vi "CommandLine.vi"() -> ()   [LabVIEW 2009]
doc: "This example shows how to use Command Line Arguments property node to launch a LabVIEW VI and pass user-defined arguments.\n\nUse the following syntax in the Command Line to launch this VI:\n\n\"<full path to LabVIEW directory>\\labview.exe\" \"<full path to LabVIEW directory>\\examples\\viserver\\cmdline.llb\\CommandLine.vi\"\n\nThis will launch CommandLine.vi\n\nThis VI is set to run when opened.\n\nAfter the VI name, enter two hyphens (--) surrounded by spaces before the user-defined arguments. \n\nThe arguments will be displayed in the front panel indicators.\n\nThe correct syntax for arguments that can be passed is\n/number:\n/boolean:\n/string:\nAfter (:) enter the appropriate value; a number, 0 or 1 boolean, a string.\n\nIf you enter more than one argument, they need to be separated with a space."
uses:
  <vilib>/Utility/miscctls.llb/LVRectTypeDef.ctl
panel:
  out "Command Line Arguments":string[](array[string])
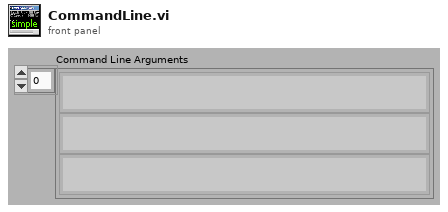
[diagram p1: front panel]
types:
  T1 = typedef "LVRectTypeDef.ctl" = cluster{"Left":i16, "Top":i16, "Right":i16, "Bottom":i16}
  T2 = enum16{"big-endian, network order", "native, host order", "little-endian"}
  T3 = enum16{"open", "replace", "create", "open or create", "replace or create", "replace or create with confirmation"}
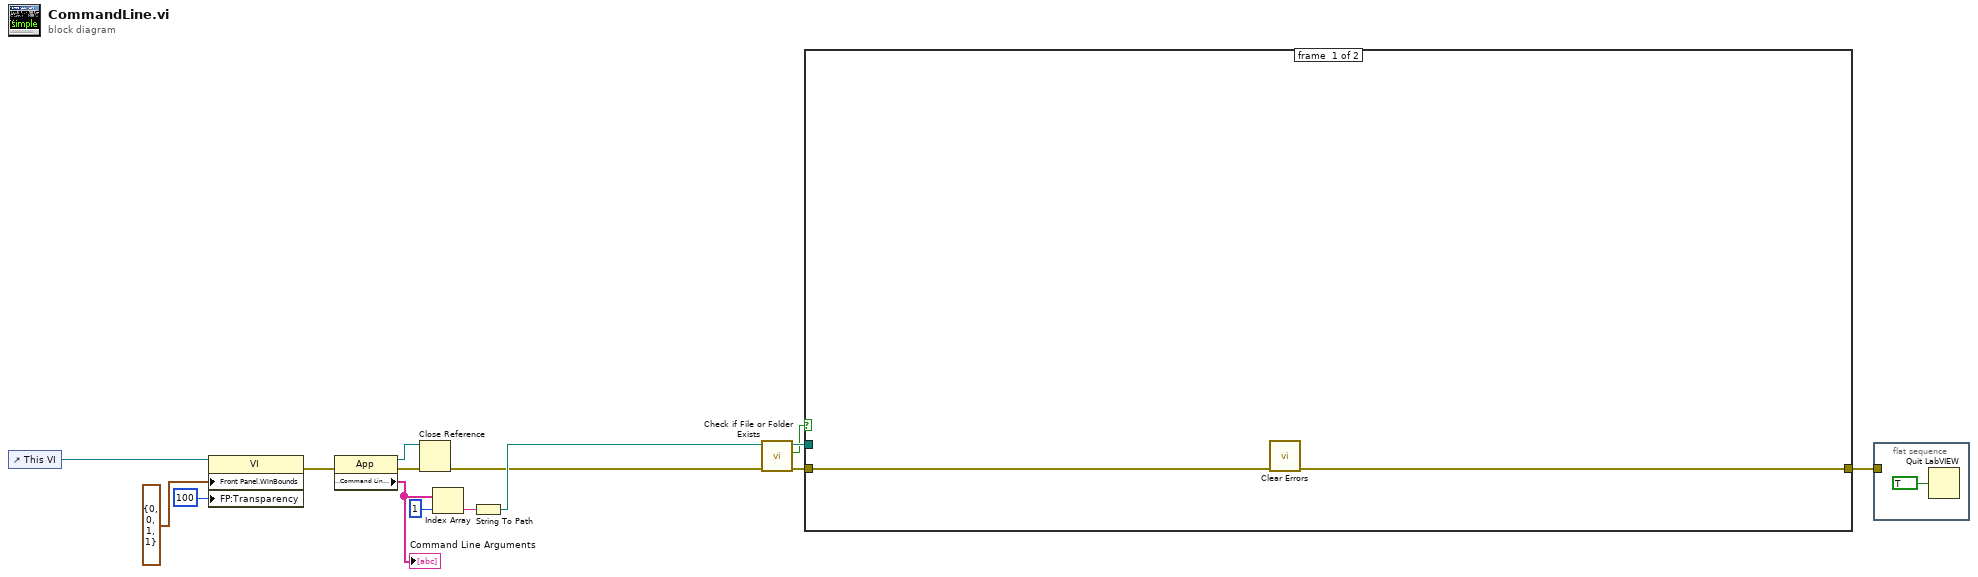
[diagram p0: block diagram]
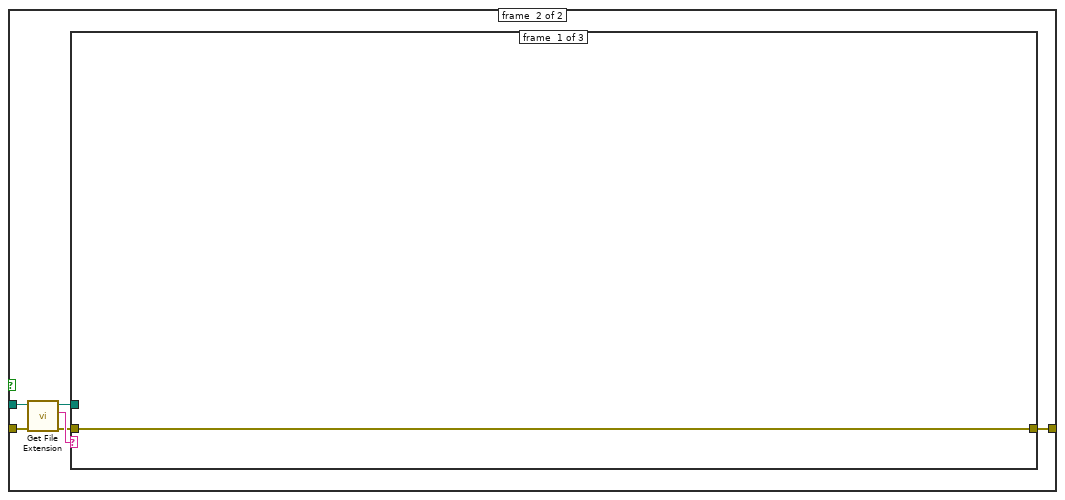
[diagram p2: hidden frame]
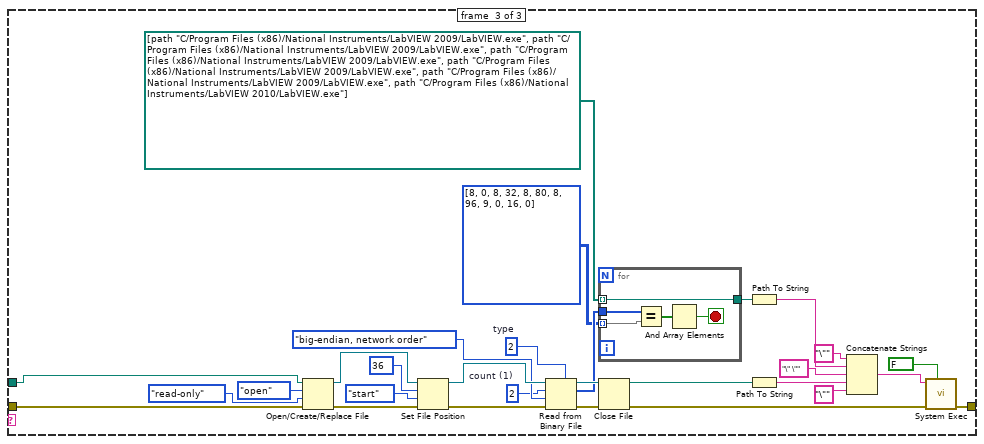
[diagram p4: hidden frame]
diagram:
  n1 = control-ref of="This VI"() -> (w10:refnum<vi>)
  n2 = property class="VI"(reference=w10, "Front Panel.WinBounds"=T1 {"Left"=0, "Top"=0, "Right"=1, "Bottom"=1} ("Front Panel Window:Window Bounds"), "FP:Transparency"=u8 100 ("Front Panel Window:Transparency")) -> (error out=w9:errorcluster)  [unwired: 1 in, 1 out]
  n3 = property class="App"(error in=w9) -> (reference out=w6:refnum<vi>, error out=w7:errorcluster, "Application:Command Line Arguments"=w5:string[])  [unwired: 1 in]
  "Command Line Arguments" <- w5
  n4 = Close Reference(reference=w6, error in (no error)=w7) -> (error out=w12:errorcluster)
  n5 = Index Array(array=w5, index=1) -> (element=w3:string)
  n6 = String To Path(string=w3) -> (path=w15:path)
  n7 = call <vilib>:"Check if File or Folder Exists.vi"("error in (no error)"=w12, "path"=w15) -> ("error out"=w11:errorcluster, "file or folder exists?"=w13:bool, "dup path"=w14:path)  [unwired: 7 in]
  n8 = case shown="True" w13 {
    tunnel: w14 -> [_ w21]
    tunnel: w11 -> [w17 w20]
    tunnel: [w16 w18] -> w8
    frame #0 {
      n9 = call <vilib>:"Clear Errors.vi"("error in (no error)"=w17) -> ("error out"=w16:errorcluster)  [unwired: 6 in]
    }
    frame #1 {
      n10 = call <vilib>:"Get File Extension.vi"("error in (no error)"=w20, "file"=w21) -> ("error out"=w19:errorcluster, "lowercase file extension"=w23:string, "dup file"=w22:path)  [unwired: 6 in, 1 out]
      n11 = case shown="\"vi\"" w23 {
        tunnel: w22 -> [_ _ w27]
        tunnel: w19 -> [w24 w25 w29]
        tunnel: [w24 w25 w28] -> w18
        frame #0 {
        }
        frame #1 {
        }
        frame #2 {
          w47 = u8 2  # type
          w48 = 2  # count (1)
          n12 = Open/Create/Replace File(file path (use dialog)=w27, error in=w29, operation (0:open)=T3."open", access (0:read/write)=enum16{"read/write", "read-only", "write-only"}."read-only") -> (refnum out=w52:refnum<file>, error out=w42:errorcluster)  [unwired: 2 in, 1 out]
          n13 = Set File Position(offset (in bytes) (0)=i64 36, refnum=w52, from (0:start)=enum16{"start", "end", "current"}."start", error in=w42) -> (refnum out=w50:refnum<file>, error out=w45:errorcluster)
          n14 = Read from Binary File(5:w47, 8:w45, 9:T2."big-endian, network order" ("byte order (0:big-endian, network order)"), 10:w48, 11:w50) -> (0:w46:errorcluster, 2:w41:u8[], 3:w44:refnum<file>)  [unwired: 1 in, 1 out]
          n15 = for {
            tunnel: w41 -> [w59]
            tunnel: u8[][] [[8, 0], [8, 32], [8, 80], [8, 96], [9, 0], [16, 0]] ("data 2") -> [w58] mode=indexing
            tunnel: path[] [path "C:/Program Files (x86)/National Instruments/LabVIEW 2009/LabVIEW.exe", path "C:/Program Files (x86)/National Instruments/LabVIEW 2009/LabVIEW.exe", path "C:/Program Files (x86)/National Instruments/LabVIEW 2009/LabVIEW.exe", path "C:/Program Files (x86)/National Instruments/LabVIEW 2009/LabVIEW.exe", path "C:/Program Files (x86)/National Instruments/LabVIEW 2009/LabVIEW.exe", path "C:/Program Files (x86)/National Instruments/LabVIEW 2010/LabVIEW.exe"] ("Array") -> [w56] mode=indexing
            tunnel: [w56] -> w38
            stop <- w55 stop-if-true
            n16 = Equal?(x=w59, y=w58) -> (x = y?=w57:bool[])
            n17 = And Array Elements(Boolean array=w57) -> (logical AND=w55:bool)
          }
          n18 = Close File(refnum=w44, error in=w46) -> (path=w26:path, error out=w30:errorcluster)
          n19 = Path To String(path=w38) -> (string=w37:string)
          n20 = Path To String(path=w26) -> (string=w34:string)
          n21 = Concatenate Strings("\"" ("string"), w37, "\" \"" ("string"), w34, "\"" ("string")) -> (w32:string)
          n22 = call <vilib>:"System Exec.vi"("wait until completion? (T)"=FALSE, "error in (no error)"=w30, "command line"=w32) -> ("error out"=w28:errorcluster)  [unwired: 5 in, 3 out]
        }
      }
    }
  }
  n23 = flat-sequence {
    tunnel: w8 -> [_]
    frame #0 {
      n24 = Quit LabVIEW(quit? (T)=TRUE) -> ()
    }
  }
